vi "globe.vi"() -> ()   [LabVIEW 2014]
panel:
  out "ret_ok":bool
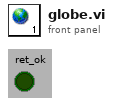
[diagram p1: front panel]
diagram:
